vi "PROVA CLIENT.vi"() -> ()   [LabVIEW 2016]
uses:
  Pedrollo Server/TypeDef/IN_Cluster.ctl
  Pedrollo Server/TypeDef/OUT_CLUSTER.ctl
panel:
  in  "Scritture":T1={"DO "=[], "AO"=[0.004], "Scelta banco PC1"=0.0, "Scelta banco PC2"=0.0, "Scelta ASP PC1"=0.0, "Scelta ASP PC2"=0.0, "Scelta MAND PC1"=0.0, "Scelta MAND PC2"=0.0, "Scelta Q PC1"=0.0, "Scelta Q PC2"=0.0} {"AO" format="%f%0.2f"}
  in  "stop":bool
  out "IN CLUSTER":T2 {"Stato uscite"."AO" format="%f%0.2f"; "AI2" format="%#_6f"; "TC" format="%#_4f"; "AI1" format="%#_6f"}
  # "prova client"
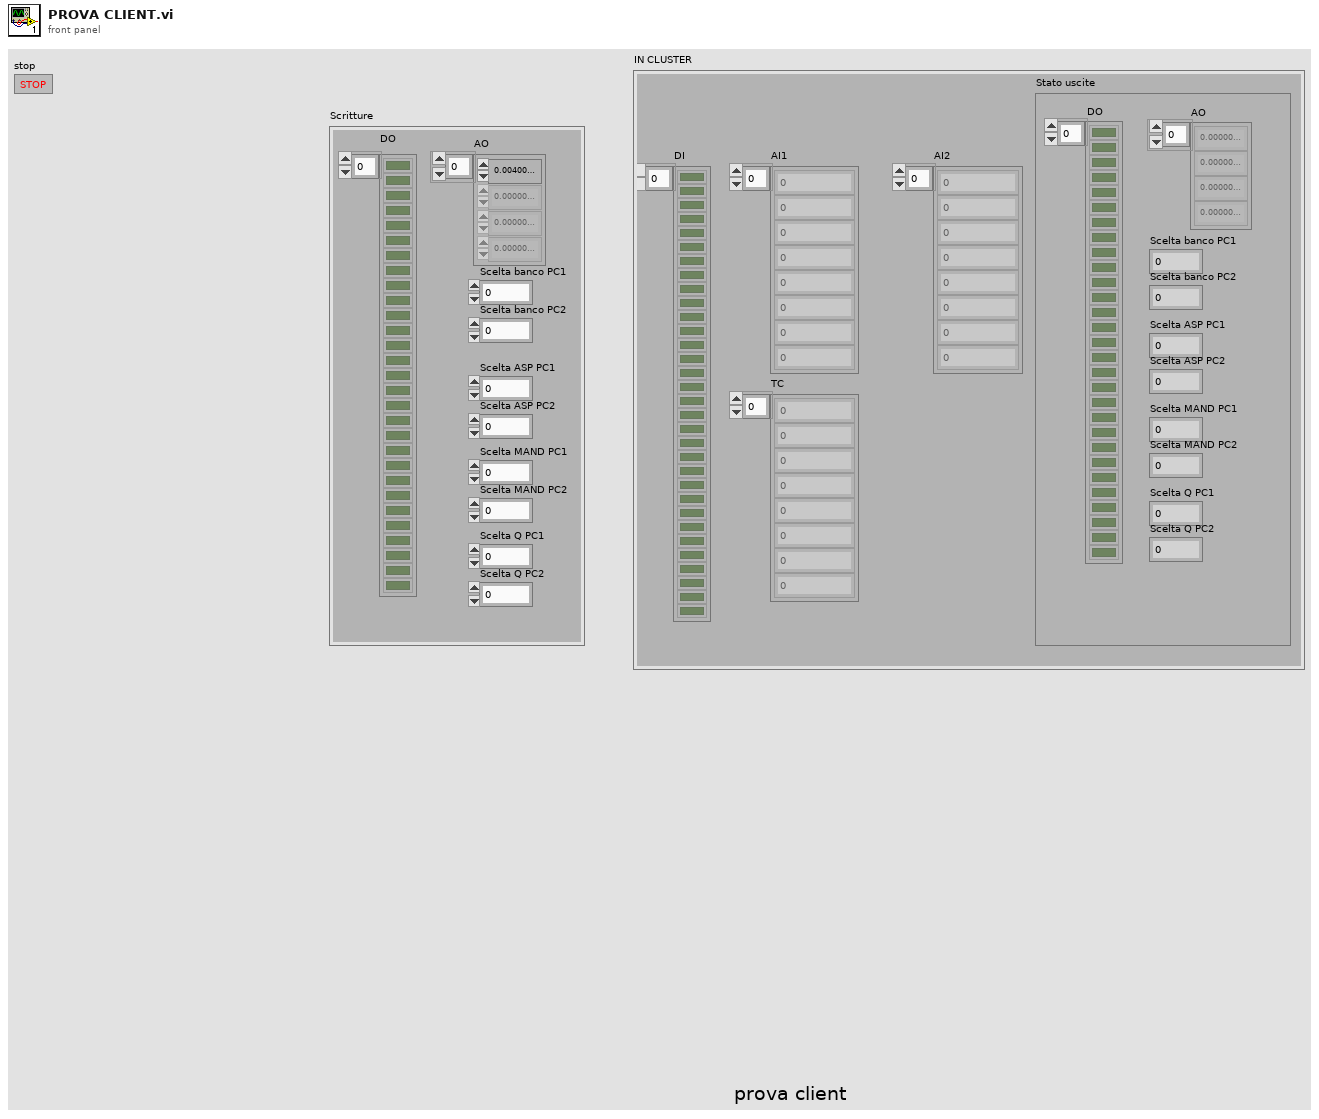
[diagram p1: front panel]
types:
  T1 = typedef "OUT_CLUSTER.ctl" = cluster{"DO ":bool[], "AO":dbl[], "Scelta banco PC1":dbl, "Scelta banco PC2":dbl, "Scelta ASP PC1":dbl, "Scelta ASP PC2":dbl, "Scelta MAND PC1":dbl, "Scelta MAND PC2":dbl, "Scelta Q PC1":dbl, "Scelta Q PC2":dbl}
  T2 = typedef "IN_Cluster.ctl" = cluster{"DI":bool[], "AI1":dbl[], "TC":dbl[], "AI2":dbl[], "Stato uscite":T1}
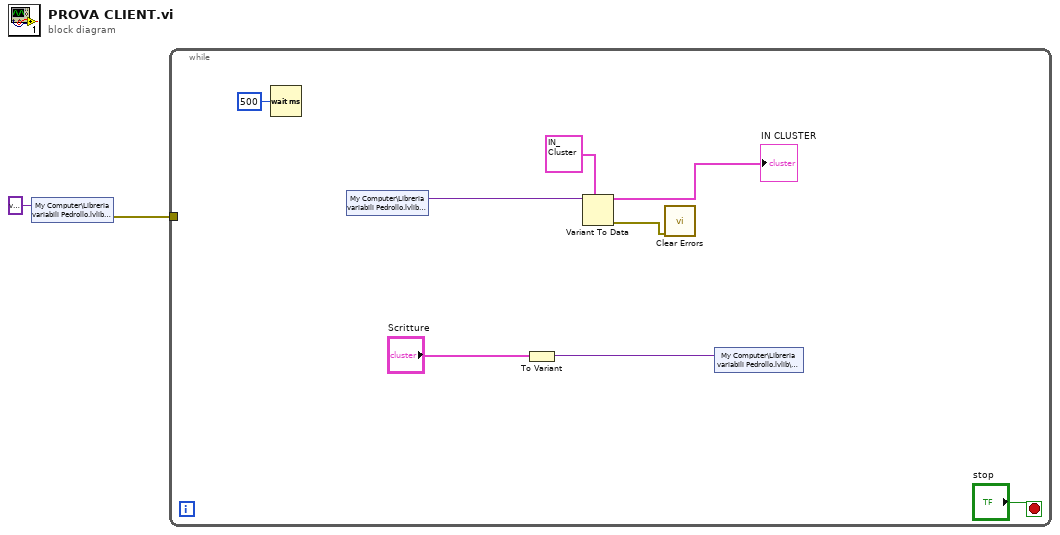
[diagram p0: block diagram]
diagram:
  n1 = shared-variable "My Computer\\Libreria variabili Pedrollo.lvlib\\Letture"(variant ("Letture")) -> (error out=w2:errorcluster)  [unwired: 1 in]
  n2 = while {
    tunnel: w2 -> [_]
    stop <- "stop" stop-if-true
    n3 = Wait (ms)(milliseconds to wait=u32 500) -> ()  [unwired: 1 out]
    n4 = shared-variable "My Computer\\Libreria variabili Pedrollo.lvlib\\Letture"() -> (w5:variant)  [unwired: 1 in, 1 out]
    n5 = To Variant(anything="Scritture") -> (Variant=w3:variant)
    n6 = Variant To Data(type=T2 {"DI"=[], "AI1"=[], "TC"=[], "AI2"=[], "Stato uscite"={"DO "=[], "AO"=[], "Scelta banco PC1"=0.0, "Scelta banco PC2"=0.0, "Scelta ASP PC1"=0.0, "Scelta ASP PC2"=0.0, "Scelta MAND PC1"=0.0, "Scelta MAND PC2"=0.0, "Scelta Q PC1"=0.0, "Scelta Q PC2"=0.0}} ("IN CLUSTER"), Variant=w5) -> (data=→"IN CLUSTER":T2, error out=w6:errorcluster)  [unwired: 1 in]
    n7 = call <vilib>:"Clear Errors.vi"("error in (no error)"=w6) -> ()  [unwired: 5 in, 2 out]
    n8 = shared-variable "My Computer\\Libreria variabili Pedrollo.lvlib\\Scritture"(w3) -> ()  [unwired: 1 in, 1 out]
  }
